vi "ultrasonic PING.vi"(7 "DIO Refnum":refnum<k21>, 8 "DIR":bool, 9 "OUT":bool, 10 "timeout(us)":i32, 11 "F selection":bool) -> (1 "IN":bool, 3 "ultrasonic output":i32)   [LabVIEW 2019]
uses:
  <vilib>/rvi/eio/common/nirviEmuTemplateMethod_errors.vi
  <vilib>/eio/EIOMethodNode/EIOMethodNode.xnode
  <vilib>/eio/EIONode/EIONode.xnode
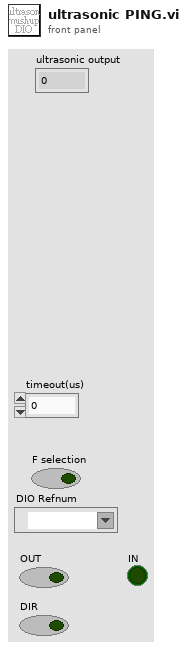
[diagram p1: front panel]
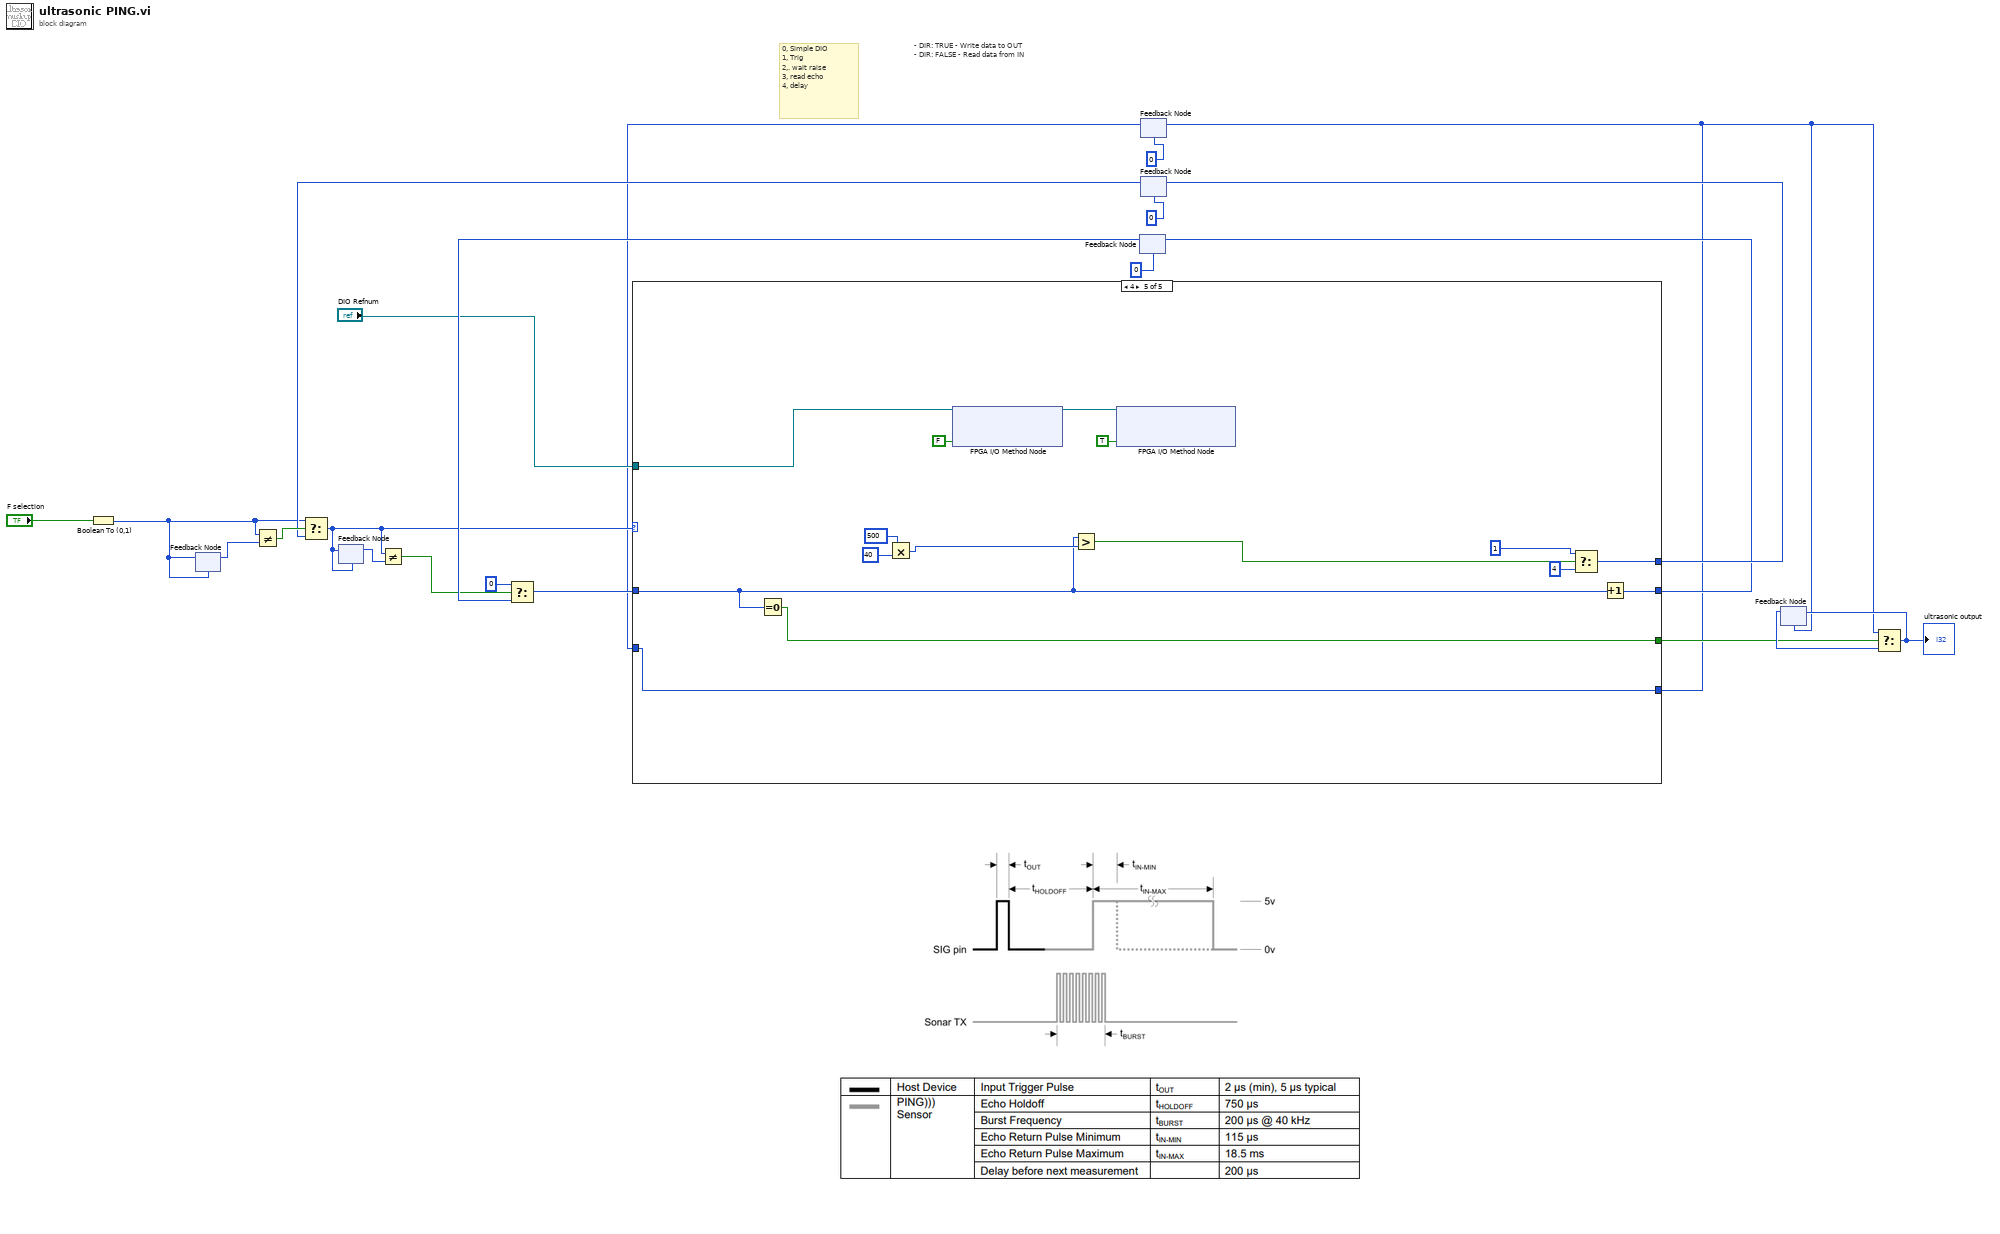
[diagram p0: block diagram]
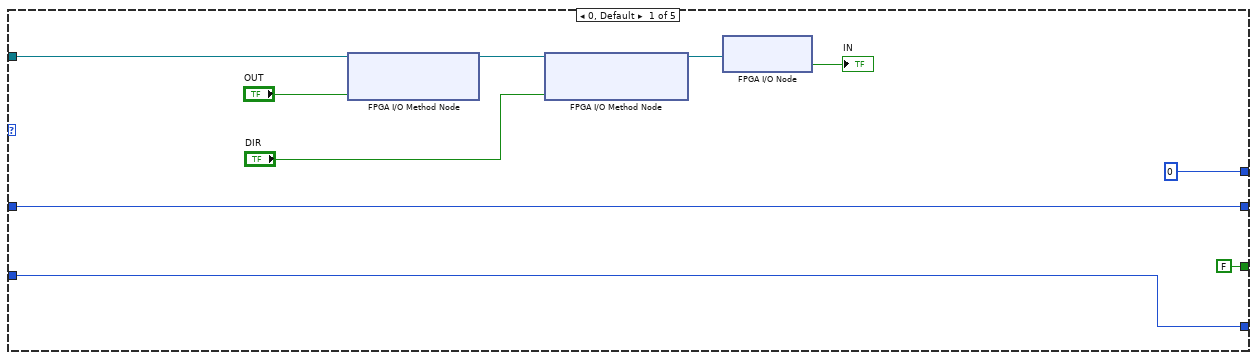
[diagram p2: hidden frame]
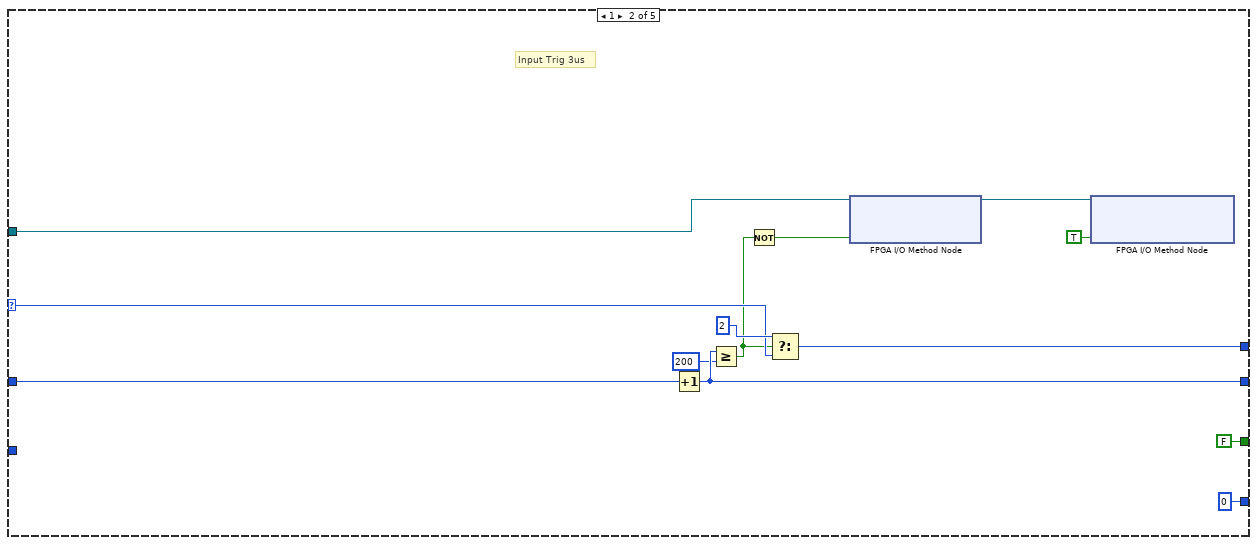
[diagram p3: hidden frame]
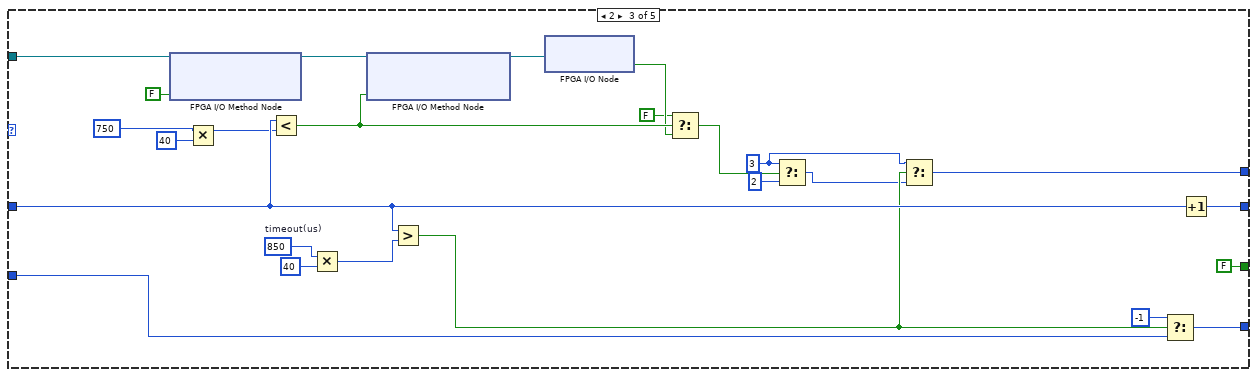
[diagram p4: hidden frame]
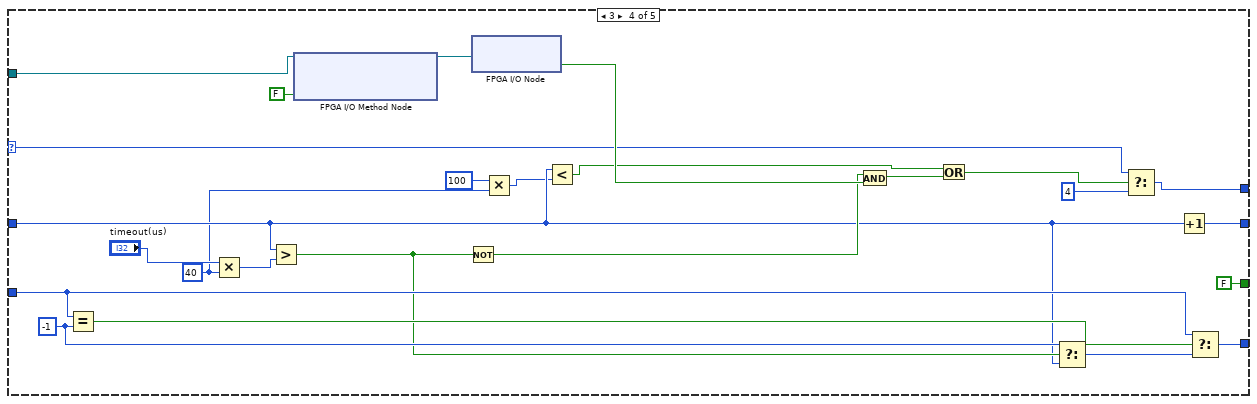
[diagram p5: hidden frame]
diagram:
  # "- DIR: TRUE - Write data to OUT\n- DIR: FALSE - Read data from IN"
  # "0, Simple DIO\n1, Trig\n2,. wait raise\n3, read echo\n4, delay"
  n1 = Boolean To (0,1)(Boolean="F selection") -> (0, 1=w5:i16)
  n2 = feedback-in #1(w5) -> ()
  n3 = feedback #1(w5) -> (w20:i16)
  n4 = Not Equal?(x=w5, y=w20) -> (x != y?=w19:bool)
  n5 = feedback #2(0) -> (w16:i32)
  n6 = feedback #3(0) -> (w6:i32)
  n7 = feedback #4(i16 0) -> (w8:i16)
  n8 = Select(t=w5, s=w19, f=w8) -> (s? t:f=w14:i16)
  n9 = feedback-in #5(w14) -> ()
  n10 = feedback #5(w14) -> (w13:i16)
  n11 = Not Equal?(x=w14, y=w13) -> (x != y?=w12:bool)
  n12 = Select(t=0, s=w12, f=w16) -> (s? t:f=w15:i32)
  n13 = case shown="4" w14 {
    selector: w14 -> [_ w40 _ w88 _]
    tunnel: [i16 0 w44 w49 w90 w106] -> w21
    tunnel: w15 -> [w24 w45 w55 w76 w98]
    tunnel: [w24 w42 w62 w92 w110] -> w10
    tunnel: "DIO Refnum" -> [w26 w38 w68 w94 w100]
    tunnel: w6 -> [w25 _ w57 w85 w97]
    tunnel: [w25 0 ("t") w56 w87 w97] -> w1
    tunnel: [FALSE FALSE FALSE FALSE w96] -> w2
    frame 0, Default {
      n14 = xnode "FPGA I/O Method Node"("FPGA I/O In"=w26, "Data"="OUT") -> ("FPGA I/O Out"=w29:refnum<k21>)
      n15 = xnode "FPGA I/O Method Node"("FPGA I/O In"=w29, "Enable"="DIR") -> ("FPGA I/O Out"=w28:refnum<k21>)
      n16 = xnode "FPGA I/O Node"("FPGA I/O In"=w28) -> ("I/O Item"=→"IN":bool)  [unwired: 1 out]
    }
    frame 1 {
      # "Input Trig 3us"
      n17 = Increment(x=w45) -> (x+1=w42:i32)
      n18 = Greater Or Equal?(x=w42, y=200) -> (x >= y?=w37:bool)
      n19 = Not(x=w37) -> (.not. x?=w35:bool)
      n20 = Select(t=i16 2, s=w37, f=w40) -> (s? t:f=w44:i16)
      n21 = xnode "FPGA I/O Method Node"("FPGA I/O In"=w38, "Data"=w35) -> ("FPGA I/O Out"=w39:refnum<k21>)
      n22 = xnode "FPGA I/O Method Node"("FPGA I/O In"=w39, "Enable"=TRUE) -> ()  [unwired: 1 out]
    }
    frame 2 {
      w59 = 850  # timeout(us)
      w51 = i16 3
      n23 = xnode "FPGA I/O Method Node"("FPGA I/O In"=w68, "Data"=FALSE) -> ("FPGA I/O Out"=w70:refnum<k21>)
      n24 = Multiply(x=750 ("y"), y=40) -> (x*y=w48:i32)
      n25 = Less?(x=w55, y=w48) -> (x < y?=w65:bool)
      n26 = Multiply(x=w59, y=40) -> (x*y=w54:i32)
      n27 = xnode "FPGA I/O Method Node"("FPGA I/O In"=w70, "Enable"=w65) -> ("FPGA I/O Out"=w69:refnum<k21>)
      n28 = Greater?(x=w55, y=w54) -> (0:w52:bool)
      n29 = xnode "FPGA I/O Node"("FPGA I/O In"=w69) -> ("I/O Item"=w64:bool)  [unwired: 1 out]
      n30 = Select(t=FALSE, s=w65, f=w64) -> (s? t:f=w61:bool)
      n31 = Select(t=w51, s=w61, f=i16 2) -> (s? t:f=w50:i16)
      n32 = Select(t=w51, s=w52, f=w50) -> (s? t:f=w49:i16)
      n33 = Select(t=-1, s=w52, f=w57) -> (s? t:f=w56:i32)
      n34 = Increment(x=w55) -> (x+1=w62:i32)
    }
    frame 3 {
      w74 = 40 ("y")
      w81 = -1 ("y")
      n35 = Equal?(x=w85, y=w81) -> (x = y?=w86:bool)
      n36 = Multiply(x="timeout(us)", y=w74) -> (x*y=w83:i32)
      n37 = Greater?(x=w76, y=w83) -> (0:w80:bool)
      n38 = xnode "FPGA I/O Method Node"("FPGA I/O In"=w94, "Enable"=FALSE) -> ("FPGA I/O Out"=w95:refnum<k21>)
      n39 = Not(x=w80) -> (.not. x?=w79:bool)
      n40 = xnode "FPGA I/O Node"("FPGA I/O In"=w95) -> ("I/O Item"=w89:bool)  [unwired: 1 out]
      n41 = Multiply(x=100, y=w74) -> (x*y=w75:i32)
      n42 = Less?(x=w76, y=w75) -> (x < y?=w72:bool)
      n43 = And(x=w79, y=w89) -> (x .and. y?=w78:bool)
      n44 = Or(x=w72, y=w78) -> (x .or. y?=w77:bool)
      n45 = Select(t=w81, s=w80, f=w76) -> (s? t:f=w82:i32)
      n46 = Select(t=w88, s=w77, f=i16 4) -> (s? t:f=w90:i16)
      n47 = Increment(x=w76) -> (x+1=w92:i32)
      n48 = Select(t=w85, s=w86, f=w82) -> (s? t:f=w87:i32)
    }
    frame 4 {
      n49 = Equal To 0?(x=w98) -> (x = 0?=w96:bool)
      n50 = Multiply(x=500, y=40) -> (x*y=w107:i32)
      n51 = xnode "FPGA I/O Method Node"("FPGA I/O In"=w100, "Data"=FALSE) -> ("FPGA I/O Out"=w102:refnum<k21>)
      n52 = Greater?(x=w98, y=w107) -> (0:w105:bool)
      n53 = xnode "FPGA I/O Method Node"("FPGA I/O In"=w102, "Enable"=TRUE) -> ()  [unwired: 1 out]
      n54 = Select(t=i16 1, s=w105, f=i16 4) -> (s? t:f=w106:i16)
      n55 = Increment(x=w98) -> (x+1=w110:i32)
    }
  }
  n56 = feedback-in #2(w10) -> ()
  n57 = feedback-in #3(w1) -> ()
  n58 = feedback-in #4(w21) -> ()
  n59 = feedback #6(w1) -> (w4:i32)
  n60 = Select(t=w1, s=w2, f=w4) -> (s? t:f=w3:i32)
  "ultrasonic output" <- w3
  n61 = feedback-in #6(w3) -> ()
